vi "ke37xx Configure DAC Channel Mode.vi"(8 "error in (no error)":errorcluster, 9 "Mode (Protected Voltage 1)":T1(ring)=enum."Protected Voltage 1", 10 "DAC Channels":string, 11 "VISA Resource Name":refnum<visa-resource-name>) -> (0 "error out":errorcluster, 3 "VISA Resource Name Out":refnum<visa-resource-name>)   [LabVIEW 2009, in "Keithley 3700 Series.lvlib"]
doc: "This VI sets the DAC to output current or voltage."
uses:
  <instrlib>/Keithley 3706/Keithley 3700 Series.lvlib
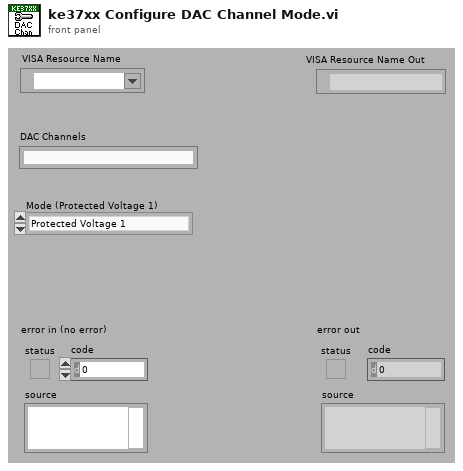
[diagram p1: front panel]
types:
  T1 = enum16{"Voltage 1", "Current 1", "Current 2", "Protected Voltage 1", "Protected Current 1", "Protected Current 2"}
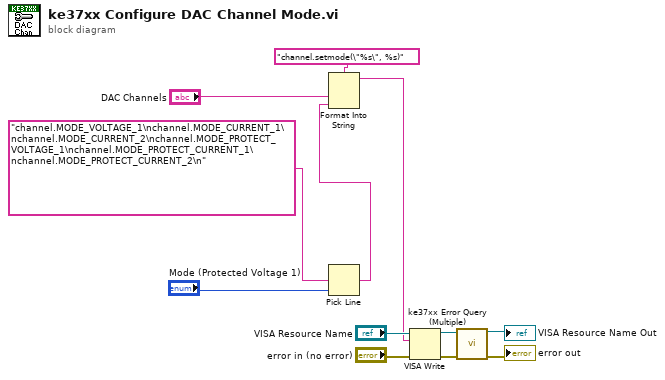
[diagram p0: block diagram]
diagram:
  n1 = Pick Line(multi-line string="channel.MODE_VOLTAGE_1\nchannel.MODE_CURRENT_1\nchannel.MODE_CURRENT_2\nchannel.MODE_PROTECT_VOLTAGE_1\nchannel.MODE_PROTECT_CURRENT_1\nchannel.MODE_PROTECT_CURRENT_2\n", line index="Mode (Protected Voltage 1)") -> (output string=w3:string)  [unwired: 1 out]
  n2 = Format Into String(format string="channel.setmode(\"%s\", %s)", "DAC Channels", w3) -> (resulting string=w7:string)  [unwired: 2 in, 1 out]
  n3 = VISA Write(VISA resource name="VISA Resource Name", write buffer=w7, error in (no error)="error in (no error)") -> (VISA resource name out=w6:refnum<visa-resource-name>, error out=w5:errorcluster)  [unwired: 1 out]
  n4 = call <instrlib>:"ke37xx Error Query (Multiple).vi"("VISA resource name"=w6, "error in (no error)"=w5) -> ("VISA resource name out"=→"VISA Resource Name Out":refnum<visa-resource-name>, "error out"=→"error out":errorcluster)  [unwired: 12 out]
